vi "NotifyObserver_Container.vi"(8 "error in":errorcluster, 9 "ObservableDataValue":variant, 10 "ObservableDataName":string, 11 "IstanceName":string) -> (0 "error out":errorcluster)   [LabVIEW 2025, in "ObserverClass.lvlib"]
doc: "Send Notification to all the Observer"
uses:
  ObserverClass.lvlib
  ObserverClass/Controls/observerControl.ctl
  ObserverClass/ObserverClass.lvclass
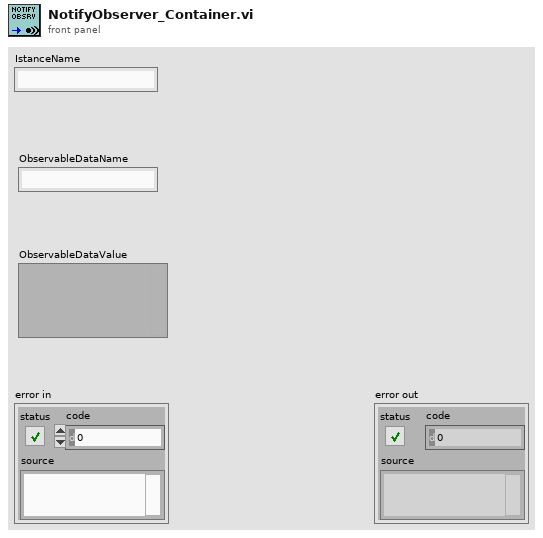
[diagram p1: front panel]
types:
  T1 = enum16{"Get", "Set", "Init", "Remove", "Destroy"}
  T2 = typedef "ObserverClass.lvlib/ObserverClass.lvclass/observerControl.ctl" = cluster{"ObservableName":string, "ObservableValue":variant, "SenderName":string}
  T3 = map{string, cluster{"ObserverEvent":refnum<user-event>, "ObserverNr":u64, "Value":variant}}
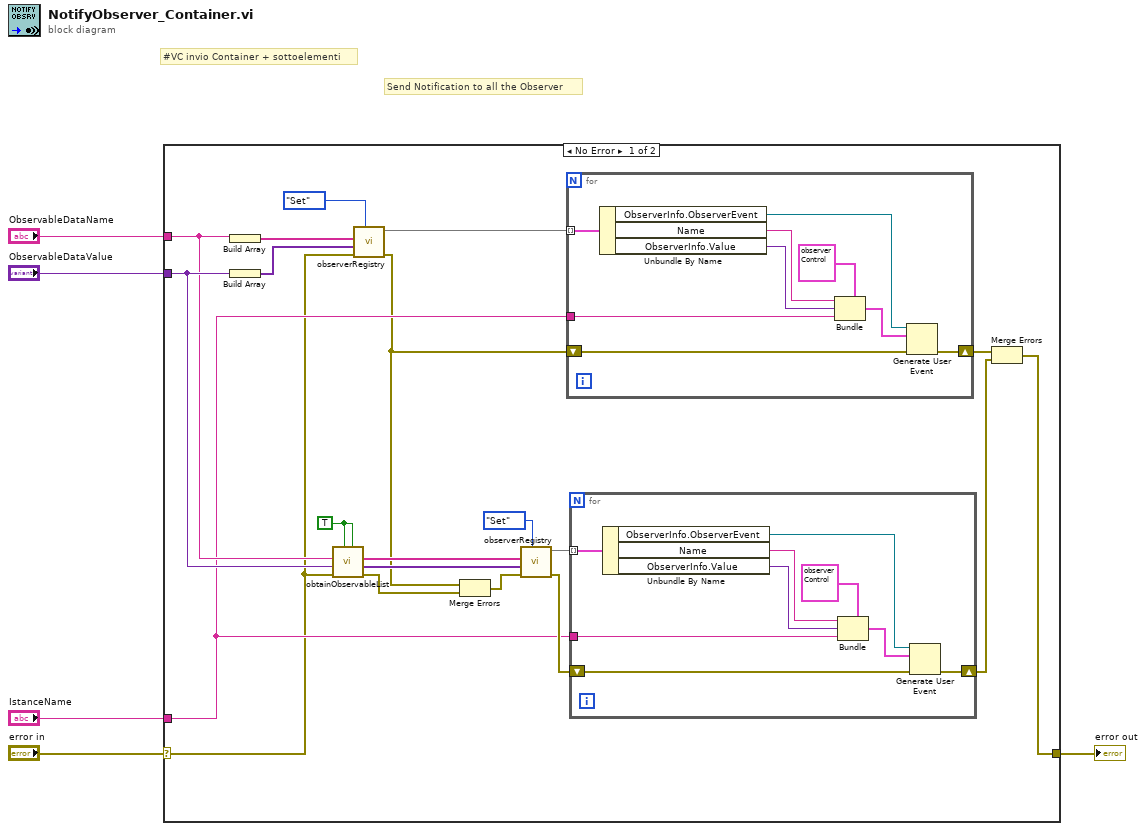
[diagram p0: block diagram]
diagram:
  # "#VC invio Container + sottoelementi"
  # "Send Notification to all the Observer"
  n1 = case shown="No Error" "error in" {
    selector: "error in" -> [w8 w44]
    tunnel: "ObservableDataName" -> [w19 _]
    tunnel: "ObservableDataValue" -> [w20 _]
    tunnel: "IstanceName" -> [w13 _]
    tunnel: [w15 w44] -> w5
    frame No Error {
      w12 = TRUE ("AllHierarchy (T)")
      n2 = Build Array(w19) -> (w22:string[])
      n3 = Build Array(w20) -> (w21:variant[])
      n4 = call "obtainObservableList.vi"("ExplodeContainer (F)"=w12, "AllHierarchy (T)"=w12, "error in"=w8, "ObservableData"=w20, "ObservableName"=w19) -> ("error out"=w9:errorcluster, "ObservableValue"=w10:variant[], "ObservableName"=w11:string[])  [unwired: 4 in]
      n5 = call "observerRegistry.vi"("Action"=T1."Set", "error in"=w8, "ObservableValue"=w21, "ObservableName"=w22) -> ("error out"=w6:errorcluster, "Observable out"=w24:T3)  [unwired: 5 in, 1 out]
      n6 = Merge Errors(w6, w9) -> (w7:errorcluster)
      n7 = call "observerRegistry.vi"("Action"=T1."Set", "error in"=w7, "ObservableValue"=w10, "ObservableName"=w11) -> ("error out"=w18:errorcluster, "Observable out"=w17:T3)  [unwired: 5 in, 1 out]
      n8 = for {
        tunnel: w24 -> [w43] mode=indexing
        tunnel: w13 -> [w38]
        shift-right: [w35] -> w23
        shift-left: w6 -> [w36]
        n9 = Unbundle By Name(w43) -> ("ObserverInfo.ObserverEvent"=w42:refnum<user-event>, "Name"=w39:string, "ObserverInfo.Value"=w37:variant)
        n10 = Bundle(cluster=T2 {"ObservableName"="", "ObservableValue"=variant, "SenderName"=""} ("event data"), "ObservableName"=w39, "ObservableValue"=w37, "SenderName"=w38) -> (w41:T2)
        n11 = Generate User Event(user event=w42, event data cluster=w41, error in=w36) -> (error out=w35:errorcluster)  [unwired: 1 in, 1 out]
      }
      n12 = for {
        tunnel: w17 -> [w34] mode=indexing
        tunnel: w13 -> [w29]
        shift-right: [w26] -> w14
        shift-left: w18 -> [w27]
        n13 = Unbundle By Name(w34) -> ("ObserverInfo.ObserverEvent"=w33:refnum<user-event>, "Name"=w30:string, "ObserverInfo.Value"=w28:variant)
        n14 = Bundle(cluster=T2 {"ObservableName"="", "ObservableValue"=variant, "SenderName"=""} ("event data"), "ObservableName"=w30, "ObservableValue"=w28, "SenderName"=w29) -> (w32:T2)
        n15 = Generate User Event(user event=w33, event data cluster=w32, error in=w27) -> (error out=w26:errorcluster)  [unwired: 1 in, 1 out]
      }
      n16 = Merge Errors(w23, w14) -> (w15:errorcluster)
    }
    frame Error {
    }
  }
  "error out" <- w5
